vi "CRCL Globals.vi"() -> ()   [LabVIEW 2013]
panel:
  in  "Relative Speed":dbl
  in  "Relative Acceleration":dbl
  in  "Length Units":string="mm"
  in  "AxisUnits":string[](array[string])
  in  "Axial Speeds":dbl[](array[numeric])
  in  "acceleration":dbl
  in  "speed":dbl
  in  "Object":string
  in  "Angle Units":string="degrees"
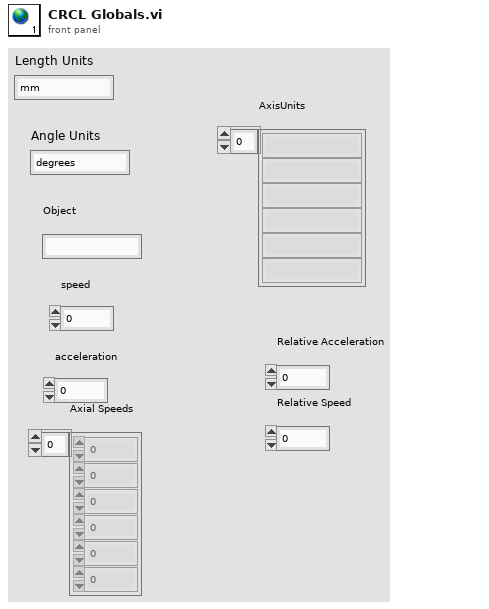
[diagram p1: front panel]
diagram:
